vi "Overlay Rectangle & Median.vi"(5 "Median End Points":cluster{"X":dbl, "Y":dbl}[](array[cluster]), 7 "Rectangle End Points":cluster{"X":dbl, "Y":dbl}[](array[cluster]), 8 "error in (no error)":errorcluster, 9 "Overlay Color":u32, 10 "Image Refunm":T2, 11 "Image Control Refnum":T1) -> (0 "error out":errorcluster)   [LabVIEW 2021, in "Image.lvlib"]
doc: "Draws a rectangle and its main axis (median) based on the coordinates of the end points provided as inputs."
uses:
  Image.lvlib
  <vilib>/vision/Image Controls.llb/IMAQ Image.ctl
  Image Control Refnum.ctl
  Error/Error.lvlib
panel:
  # "see the AlliGator License on the block diagram (Ctrl+E or Window:Show Block Diagram)"
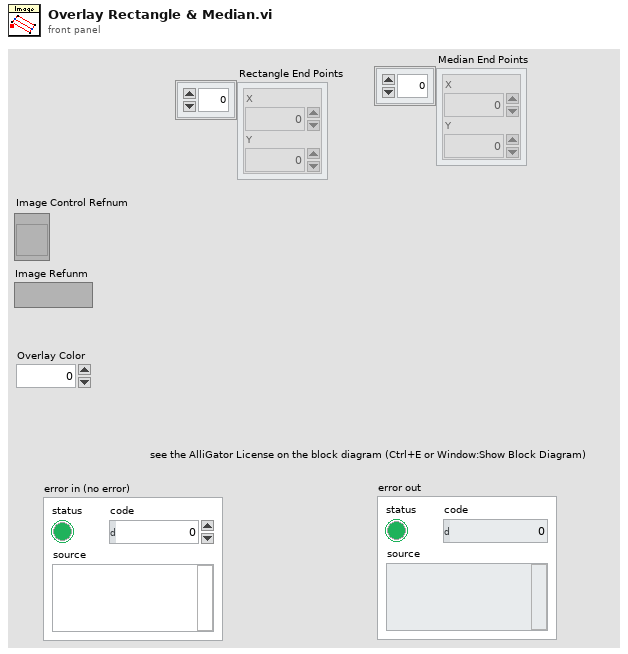
[diagram p1: front panel]
types:
  T1 = typedef "Image.lvlib/Image Control Refnum.ctl" = refnum<vi>
  T2 = typedef "IMAQ Image.ctl" = refnum<image>
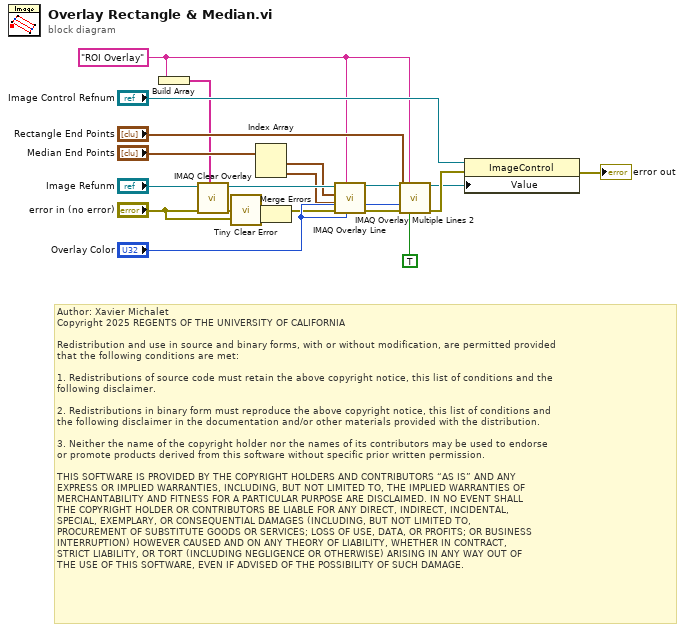
[diagram p0: block diagram]
diagram:
  w8 = "ROI Overlay" ("Groups")
  # "Author: Xavier Michalet\nCopyright 2025 REGENTS OF THE UNIVERSITY OF CALIFORNIA\n\nRedistribution and use in source and binary forms, with or without modification, are permitted provided\nthat the following conditions are met:\n\n1. Redistributions of source code must retain the above copyright notice, this list of conditions and the\nfollowing disclaimer.\n\n2. Redistributions in binary form must reproduce the above copyright notice, this list of conditions and\nthe following disclaimer in the documentation and/or other materials provided with the distribution.\n\n3. Neither the name of the copyright holder nor the names of its contributors may be used to endorse \nor promote products derived from this software without specific prior written permission.\n\nTHIS SOFTWARE IS PROVIDED BY THE COPYRIGHT HOLDERS AND CONTRIBUTORS “AS IS” AND ANY \nEXPRESS OR IMPLIED WARRANTIES, INCLUDING, BUT NOT LIMITED TO, THE IMPLIED WARRANTIES OF\nMERCHANTABILITY AND FITNESS FOR A PARTICULAR PURPOSE ARE DISCLAIMED. IN NO EVENT SHALL\nTHE COPYRIGHT HOLDER OR CONTRIBUTORS BE LIABLE FOR ANY DIRECT, INDIRECT, INCIDENTAL, \nSPECIAL, EXEMPLARY, OR CONSEQUENTIAL DAMAGES (INCLUDING, BUT NOT LIMITED TO, \nPROCUREMENT OF SUBSTITUTE GOODS OR SERVICES; LOSS OF USE, DATA, OR PROFITS; OR BUSINESS\nINTERRUPTION) HOWEVER CAUSED AND ON ANY THEORY OF LIABILITY, WHETHER IN CONTRACT, \nSTRICT LIABILITY, OR TORT (INCLUDING NEGLIGENCE OR OTHERWISE) ARISING IN ANY WAY OUT OF\nTHE USE OF THIS SOFTWARE, EVEN IF ADVISED OF THE POSSIBILITY OF SUCH DAMAGE."
  n1 = Build Array(w8) -> (w13:string[])
  n2 = call "IMAQ Clear Overlay"("Groups"=w13, "error in (no error)"="error in (no error)", "Image"="Image Refunm") -> ("error out"=w14:errorcluster, "Image Out"=w12:T2)  [unwired: 7 in]
  n3 = call "Tiny Clear Error.vi"("Error In"=w14) -> ("no Error Out"=w11:errorcluster)  [unwired: 8 in]
  n4 = Index Array(array="Median End Points") -> (element #1=w6:cluster{"X":dbl, "Y":dbl}, element #2=w5:cluster{"X":dbl, "Y":dbl})  [unwired: 2 in]
  n5 = Merge Errors(w11, "error in (no error)") -> (w2:errorcluster)
  n6 = call "IMAQ Overlay Line"("Color"="Overlay Color", "Group"=w8, "error in (no error)"=w2, "End Point"=w5, "Start Point"=w6, "Image"=w12) -> ("error out"=w10:errorcluster, "Image Out"=w7:T2)  [unwired: 4 in]
  n7 = call "IMAQ Overlay Multiple Lines 2"("Image"=w7, "Group"=w8, "Line End Points"="Rectangle End Points", "Color"="Overlay Color", "error in (no error)"=w10, "Maintain Width?"=TRUE) -> ("Image Out"=w3:T2, "error out"=w4:errorcluster)  [unwired: 8 in]
  n8 = property class="ImageControl"(reference="Image Control Refnum", error in=w4, "Value"=w3) -> (error out=→"error out":errorcluster)  [unwired: 1 out]
